vi "Handler - cRIO Health Alert.vi"(8 "error in (no error)":errorcluster, 11 "Alert Booleans":bool[](array[boolean])) -> (0 "error out":errorcluster, 3 "Exit?":bool)   [LabVIEW 2018]
uses:
  Error Handler.lvlib
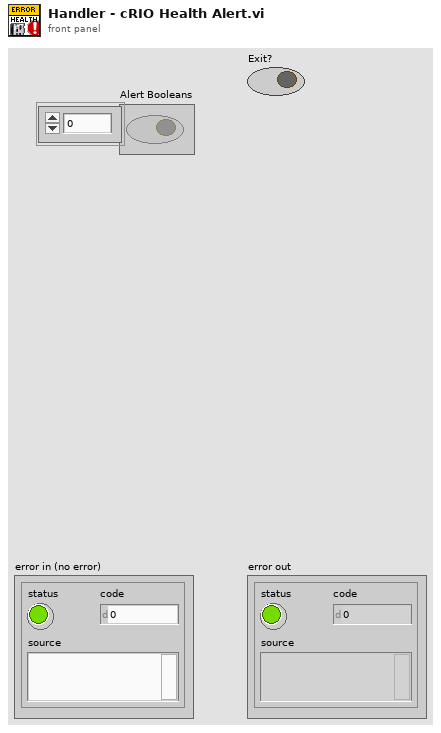
[diagram p1: front panel]
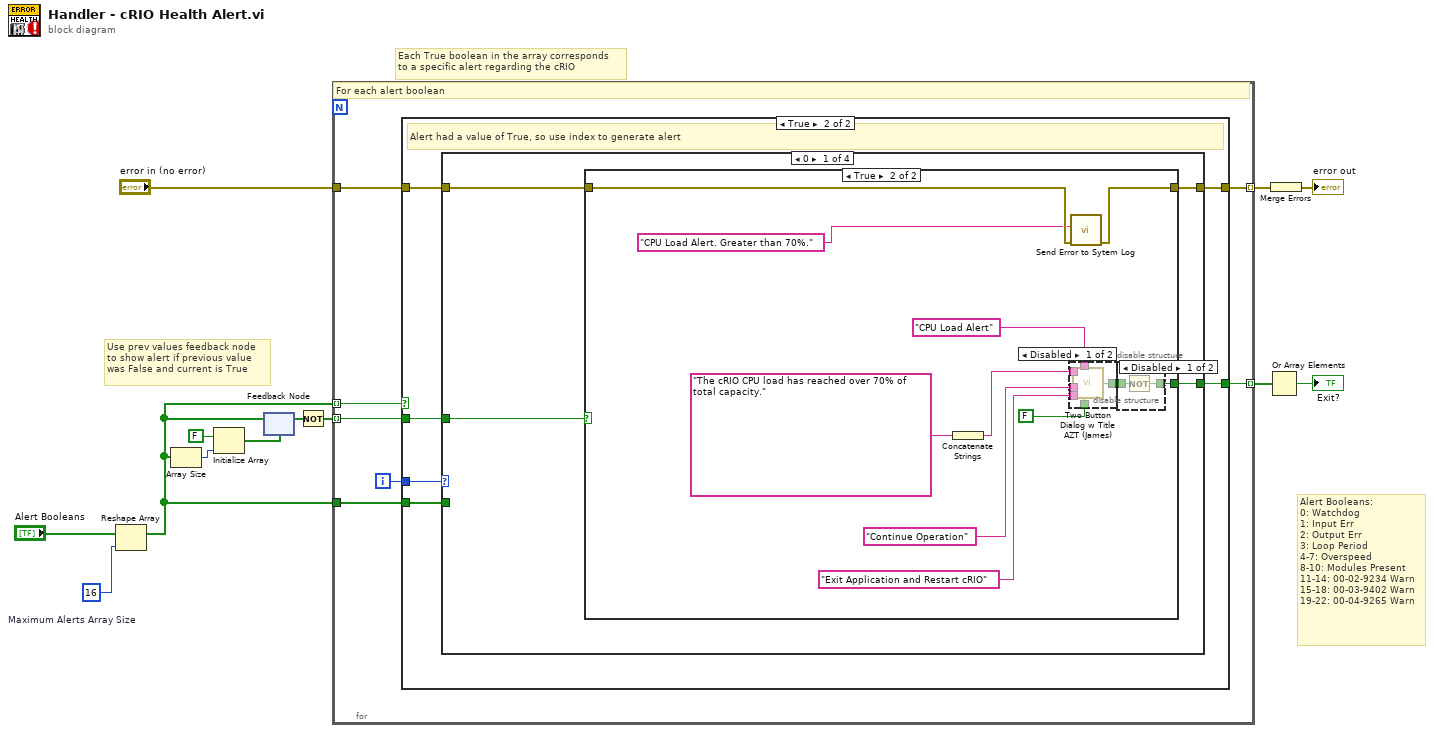
[diagram p0: block diagram]
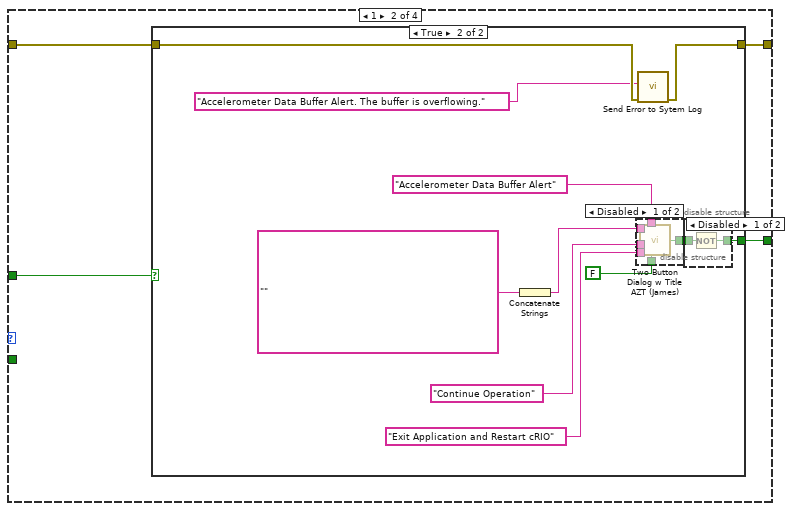
[diagram p6: hidden frame]
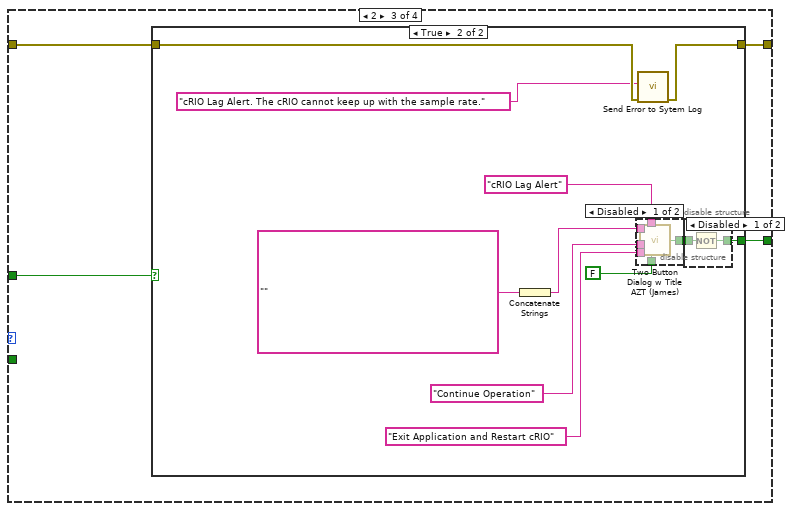
[diagram p10: hidden frame]
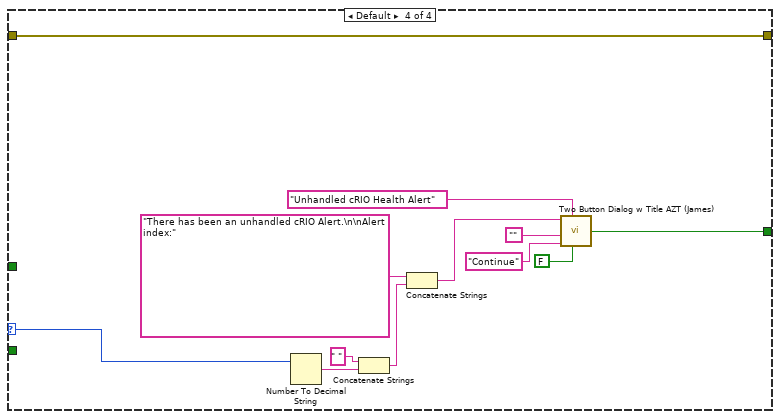
[diagram p14: hidden frame]
diagram:
  w1 = 16  # Maximum Alerts Array Size
  # "Alert Booleans:\n0: Watchdog\n1: Input Err\n2: Output Err\n3: Loop Period\n4-7: Overspeed\n8-10: Modules Present\n11-14: 00-02-9234 Warn\n15-18: 00-03-9402 Warn\n19-22: 00-04-9265 Warn"
  # "Use prev values feedback node\nto show alert if previous value\nwas False and current is True"
  # "Each True boolean in the array corresponds\nto a specific alert regarding the cRIO"
  n1 = Reshape Array("Alert Booleans", w1) -> (w2:bool[])
  n2 = Array Size(array=w2) -> (size(s)=w7:i32)
  n3 = Initialize Array(FALSE, w7) -> (w6:bool[])
  n4 = feedback #1(w6) -> (w5:bool[])
  n5 = feedback-in #1(w2) -> ()
  n6 = Not(x=w5) -> (.not. x?=w4:bool[])
  n7 = for {
    tunnel: w2 -> [w19] mode=indexing
    tunnel: "error in (no error)" -> [w17]
    tunnel: [w18] -> w10 mode=indexing
    tunnel: [w16] -> w11 mode=indexing
    tunnel: w2 -> [w15]
    tunnel: w4 -> [w14] mode=indexing
    i -> [w20]
    # "For each alert boolean"
    n8 = case shown="True" w19 {
      tunnel: w20 -> [_ w27]
      tunnel: [w21 w25] -> w18
      tunnel: w17 -> [w21 w26]
      tunnel: [_ w24] -> w16
      tunnel: w15 -> [_ w23]
      tunnel: w14 -> [_ w22]
      frame False {
      }
      frame True {
        # "Alert had a value of True, so use index to generate alert"
        n9 = case shown="0" w27 {
          selector: w27 -> [_ _ _ w102]
          tunnel: w26 -> [w29 w53 w77 w110]
          tunnel: [w28 w52 w76 w110] -> w25
          tunnel: [w31 w55 w79 w107] -> w24
          tunnel: w23 -> [_ _ _ _]
          tunnel: w22 -> [w30 w54 w78 _]
          frame 0 {
            n10 = case shown="True" w30 {
              tunnel: [_ w36] -> w31
              tunnel: w29 -> [w32 w35]
              tunnel: [w32 w34] -> w28
              frame False {
              }
              frame True {
                n11 = Concatenate Strings("The cRIO CPU load has reached over 70% of total capacity." ("message")) -> (w41:string)
                n12 = disable-structure shown="Disabled" {
                  disable-tunnel: "CPU Load Alert" ("Window Title (\"\")") -> [w51 _]
                  disable-tunnel: w41 -> [w50 _]
                  disable-tunnel: [w49 _] -> w40
                  disable-tunnel: FALSE ("Allow user to close window? (TRUE)") -> [w48 _]
                  disable-tunnel: "Exit Application and Restart cRIO" ("T button name (\"OK\")") -> [w47 _]
                  disable-tunnel: "Continue Operation" ("F button name (\"Cancel\")") -> [w46 _]
                  frame Disabled {
                    n13 = call "Two Button Dialog w Title AZT (James).vi"("Allow user to close window? (TRUE)"=w48, "Window Title (\"\")"=w51, "F button name (\"Cancel\")"=w47, "T button name (\"OK\")"=w46, "message"=w50) -> ("T Button?"=w49:bool)  [unwired: 1 in]
                  }
                  frame Enabled {
                  }
                }
                n14 = call "Send Error to Sytem Log.vi"("error in (no error)"=w35, "Error Title or Message"="CPU Load Alert. Greater than 70%." ("Window Title (\"\")")) -> ("error out"=w34:errorcluster)  [unwired: 9 in]
                n15 = disable-structure shown="Disabled" {
                  disable-tunnel: w40 -> [w45 _]
                  disable-tunnel: [w44 _] -> w36
                  frame Disabled {
                    n16 = Not(x=w45) -> (.not. x?=w44:bool)
                  }
                  frame Enabled {
                  }
                }
              }
            }
          }
          frame 1 {
            n17 = case shown="True" w54 {
              tunnel: [_ w60] -> w55
              tunnel: w53 -> [w56 w59]
              tunnel: [w56 w58] -> w52
              frame False {
              }
              frame True {
                n18 = Concatenate Strings("" ("message")) -> (w65:string)
                n19 = disable-structure shown="Disabled" {
                  disable-tunnel: "Accelerometer Data Buffer Alert" ("Window Title (\"\")") -> [w75 _]
                  disable-tunnel: w65 -> [w74 _]
                  disable-tunnel: [w73 _] -> w64
                  disable-tunnel: FALSE ("Allow user to close window? (TRUE)") -> [w72 _]
                  disable-tunnel: "Exit Application and Restart cRIO" ("T button name (\"OK\")") -> [w71 _]
                  disable-tunnel: "Continue Operation" ("F button name (\"Cancel\")") -> [w70 _]
                  frame Disabled {
                    n20 = call "Two Button Dialog w Title AZT (James).vi"("Allow user to close window? (TRUE)"=w72, "Window Title (\"\")"=w75, "F button name (\"Cancel\")"=w71, "T button name (\"OK\")"=w70, "message"=w74) -> ("T Button?"=w73:bool)  [unwired: 1 in]
                  }
                  frame Enabled {
                  }
                }
                n21 = call "Send Error to Sytem Log.vi"("error in (no error)"=w59, "Error Title or Message"="Accelerometer Data Buffer Alert. The buffer is overflowing." ("Window Title (\"\")")) -> ("error out"=w58:errorcluster)  [unwired: 9 in]
                n22 = disable-structure shown="Disabled" {
                  disable-tunnel: w64 -> [w69 _]
                  disable-tunnel: [w68 _] -> w60
                  frame Disabled {
                    n23 = Not(x=w69) -> (.not. x?=w68:bool)
                  }
                  frame Enabled {
                  }
                }
              }
            }
          }
          frame 2 {
            n24 = case shown="True" w78 {
              tunnel: [_ w84] -> w79
              tunnel: w77 -> [w80 w83]
              tunnel: [w80 w82] -> w76
              frame False {
              }
              frame True {
                n25 = Concatenate Strings("" ("message")) -> (w89:string)
                n26 = disable-structure shown="Disabled" {
                  disable-tunnel: "cRIO Lag Alert" ("Window Title (\"\")") -> [w99 _]
                  disable-tunnel: w89 -> [w98 _]
                  disable-tunnel: [w97 _] -> w88
                  disable-tunnel: FALSE ("Allow user to close window? (TRUE)") -> [w96 _]
                  disable-tunnel: "Exit Application and Restart cRIO" ("T button name (\"OK\")") -> [w95 _]
                  disable-tunnel: "Continue Operation" ("F button name (\"Cancel\")") -> [w94 _]
                  frame Disabled {
                    n27 = call "Two Button Dialog w Title AZT (James).vi"("Allow user to close window? (TRUE)"=w96, "Window Title (\"\")"=w99, "F button name (\"Cancel\")"=w95, "T button name (\"OK\")"=w94, "message"=w98) -> ("T Button?"=w97:bool)  [unwired: 1 in]
                  }
                  frame Enabled {
                  }
                }
                n28 = call "Send Error to Sytem Log.vi"("error in (no error)"=w83, "Error Title or Message"="cRIO Lag Alert. The cRIO cannot keep up with the sample rate." ("Window Title (\"\")")) -> ("error out"=w82:errorcluster)  [unwired: 9 in]
                n29 = disable-structure shown="Disabled" {
                  disable-tunnel: w88 -> [w93 _]
                  disable-tunnel: [w92 _] -> w84
                  frame Disabled {
                    n30 = Not(x=w93) -> (.not. x?=w92:bool)
                  }
                  frame Enabled {
                  }
                }
              }
            }
          }
          frame Default {
            n31 = Number To Decimal String(number=w102) -> (decimal integer string=w106:string)  [unwired: 1 in]
            n32 = Concatenate Strings(" " ("string"), w106) -> (w104:string)
            n33 = Concatenate Strings("There has been an unhandled cRIO Alert.\n\nAlert index:" ("message"), w104) -> (w108:string)
            n34 = call "Two Button Dialog w Title AZT (James).vi"("Allow user to close window? (TRUE)"=FALSE, "Window Title (\"\")"="Unhandled cRIO Health Alert" ("Window Title (\"\")"), "F button name (\"Cancel\")"="Continue" ("T button name (\"OK\")"), "T button name (\"OK\")"="", "message"=w108) -> ("T Button?"=w107:bool)  [unwired: 1 in]
          }
        }
      }
    }
  }
  n35 = Or Array Elements(Boolean array=w11) -> (logical OR=→"Exit?":bool)
  n36 = Merge Errors(w10) -> (→"error out":errorcluster)
